vi "LowPassFilter.vi"(2 "a":dbl, 3 "yf_prev":dbl, 4 "Tout":dbl) -> (0 "yf":dbl, 1 "Tout":dbl)   [LabVIEW 2023]
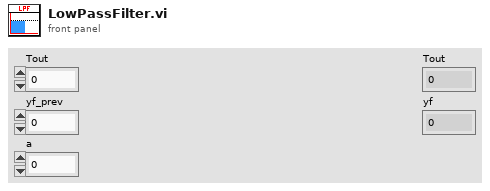
[diagram p1: front panel]
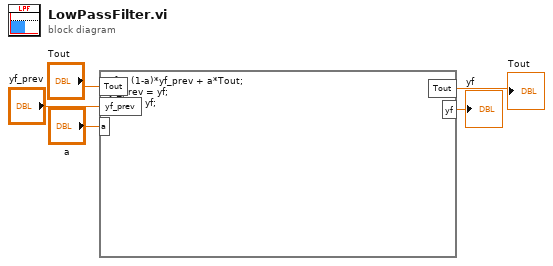
[diagram p0: block diagram]
diagram:
  n1 = formula code="yf = (1-a)*yf_prev + a*Tout;\nyf_prev = yf;\nTout = yf;"("Tout"="Tout", "yf_prev"="yf_prev", "a"="a") -> ("Tout"=→"Tout":dbl, "yf"=→"yf":dbl)
